vi "Kill Session Pin Map Service.vi"(8 "error in":errorcluster) -> (0 "error out":errorcluster)   [LabVIEW 2020, in "MeasurementServerTests.lvlib"]
uses:
  MeasurementServerTests.lvlib
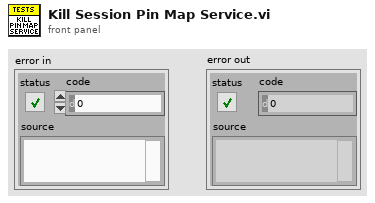
[diagram p1: front panel]
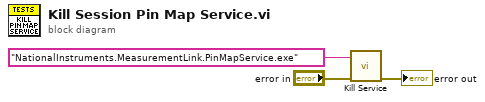
[diagram p0: block diagram]
diagram:
  n1 = call "Kill Service.vi"("error in"="error in", "full exe name"="NationalInstruments.MeasurementLink.PinMapService.exe" ("command line")) -> ("error out"=→"error out":errorcluster)  [unwired: 9 in]
